vi "Read Seats Data File.vi"(11 "Path":path) -> (3 "Array":i32[][](array[numeric]))   [LabVIEW 2019, in "flashcards.lvlib"]
uses:
  flashcards.lvlib
panel:
  out "error out":errorcluster
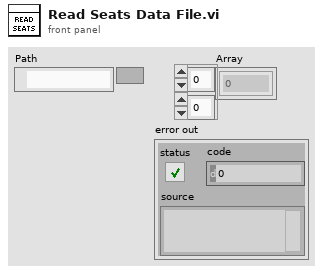
[diagram p1: front panel]
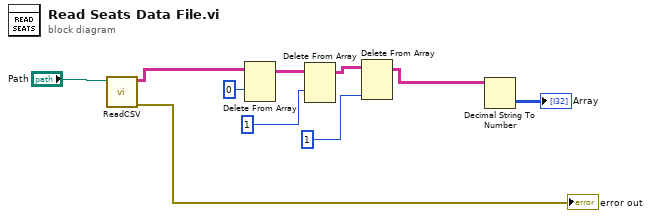
[diagram p0: block diagram]
diagram:
  n1 = call "ReadCSV.vi"("file path"="Path") -> ("error out"=→"error out":errorcluster, "Data"=w7:string[][])  [unwired: 9 in]
  n2 = Delete From Array(array=w7, index (row)=0) -> (array with subset deleted=w5:string[][])  [unwired: 2 in, 1 out]
  n3 = Delete From Array(array=w5, index (row)=1) -> (array with subset deleted=w3:string[][])  [unwired: 2 in, 1 out]
  n4 = Delete From Array(array=w3, index (col)=1 ("index (row)")) -> (array with subset deleted=w1:string[][])  [unwired: 2 in, 1 out]
  n5 = Decimal String To Number(string=w1) -> (number=→"Array":i32[][])  [unwired: 2 in, 1 out]
